vi "getOpenPort.vi"() -> (0 "port":u16)   [LabVIEW 2018]
doc: "Returns a local port not currently in use."
uses:
  <userlib>/ROS for LabVIEW Software/ROS/Code/_ROSDefinition.vi
panel:
  out "Tries":i32
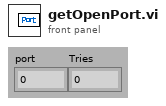
[diagram p1: front panel]
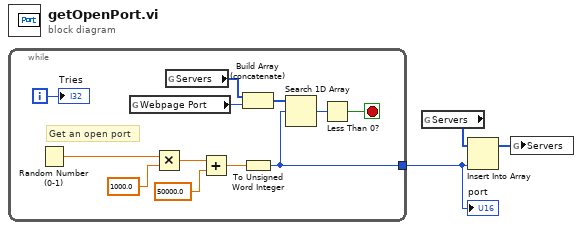
[diagram p0: block diagram]
diagram:
  n1 = while {
    tunnel: [w10] -> w3
    i -> [w8]
    stop <- w4 stop-if-true
    # "Get an open port"
    n2 = Random Number (0-1)() -> (number: 0 to 1=w14:dbl)
    n3 = global read "_ROSDefinition.vi" "Webpage Port"() -> (w6:u16)
    n4 = Multiply(x=w14, y=1000.0) -> (x*y=w13:dbl)
    n5 = global read "_ROSDefinition.vi" "Servers"() -> (w7:u16[])
    n6 = Add(x=w13, y=50000.0) -> (x+y=w11:dbl)
    n7 = Build Array (concatenate)(w7, w6) -> (w5:u16[])
    n8 = To Unsigned Word Integer(number=w11) -> (unsigned 16bit integer=w10:u16)
    n9 = Search 1D Array(1D array=w5, element=w10) -> (index of element=w9:i32)  [unwired: 1 in]
    n10 = Less Than 0?(x=w9) -> (x < 0?=w4:bool)
    "Tries" <- w8
  }
  "port" <- w3
  n11 = global read "_ROSDefinition.vi" "Servers"() -> (w2:u16[])
  n12 = Insert Into Array(array=w2, new element=w3) -> (w1:u16[])  [unwired: 1 in]
  n13 = global write "_ROSDefinition.vi" "Servers"(w1) -> ()
